vi "dotNET improvments.vi"() -> ()   [LabVIEW 2026]
uses:
  <vilib>/Utility/sysdir.llb/System Directory Type.ctl
  <vilib>/Platform/dotnet.llb/.NET Core Object To Variant.vi
  <vilib>/Platform/dotnet.llb/To .NET Core Object.vi
  C:/Program Files/dotnet/shared/Microsoft.NETCore.App/8.0.24/System.IO.FileSystem.Watcher.dll
  Program Files/dotnet/shared/Microsoft.NETCore.App/8.0.24/System.IO.FileSystem.Watcher.dll
  C:/Program Files/dotnet/shared/Microsoft.NETCore.App/8.0.24/System.Private.CoreLib.dll
  Program Files/dotnet/shared/Microsoft.NETCore.App/8.0.24/System.Private.CoreLib.dll
panel:
  out "element":string
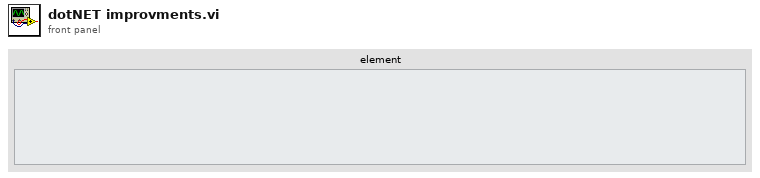
[diagram p1: front panel]
types:
  T1 = typedef "System Directory Type.ctl" = i32
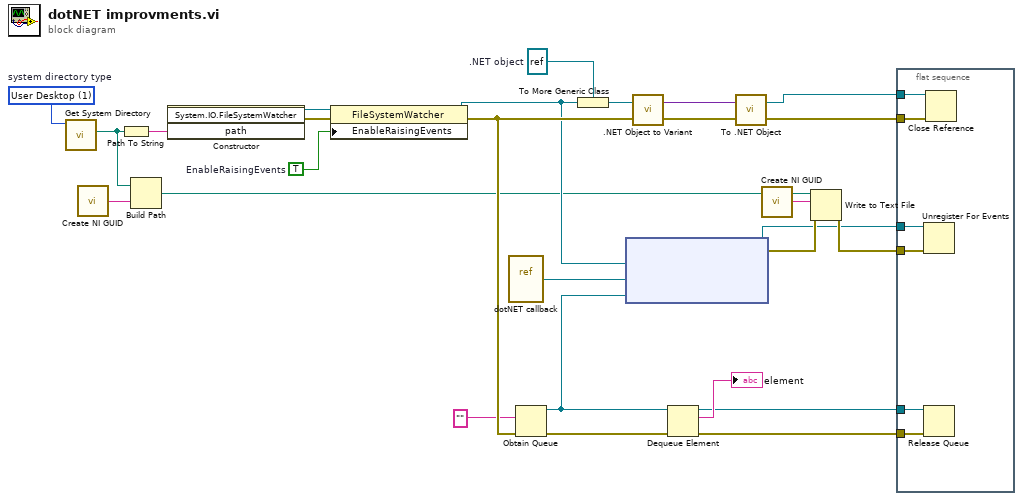
[diagram p0: block diagram]
diagram:
  w12 = refnum<k39> refnum  # .NET object
  w21 = TRUE  # EnableRaisingEvents
  w15 = T1 1 items=["User Home"=0, "User Desktop"=1, "User Documents"=2, "User Application Data"=3, "User Preferences"=4, "User Temporary"=5, "Public Documents"=6, "Public Application Data"=7, "Public Preferences"=8, "Public Cache"=13, "System Core Libraries"=9, "System Installed Libraries"=10, "Application Files"=11, "Boot Volume Root"=12]  # system directory type
  n1 = call <vilib>:"Get System Directory.vi"("system directory type"=w15) -> ("system directory"=w5:path)  [unwired: 10 in]
  n2 = call <vilib>:"Create NI GUID.vi"() -> ("NI GUID"=w6:string)
  n3 = Path To String(path=w5) -> (string=w24:string)
  n4 = Build Path(base path=w5, name or relative path=w6) -> (appended path=w4:path)
  n5 = constructor class="FileSystemWatcher"("path"=w24) -> (reference out=w23:refnum<k39>, error out=w22:errorcluster)  [unwired: 3 in, 2 out]
  n6 = property class="FileSystemWatcher"(reference=w23, error in=w22, "EnableRaisingEvents"=w21) -> (reference out=w13:refnum<k39>, error out=w25:errorcluster)
  n7 = vi-ref "dotNET callback.vi"() -> ("vi reference"=w16:refnum<vi>)
  n8 = Obtain Queue(element data type="", error in (no error)=w25) -> (queue out=w20:refnum<queue>, error out=w18:errorcluster)  [unwired: 3 in, 1 out]
  n9 = To More Generic Class(target class=w12, reference=w13) -> (generic class reference=w11:refnum<k39>)
  n10 = node(w13, w16, w20) -> (w7:refnum<k27>, w26:errorcluster)  [unwired: 2 in]
  n11 = call-poly <vilib>:".NET Object to Variant.vi"("error in (no error)"=w25, ".NET object"=w11) -> ("error out"=w9:errorcluster, "variant"=w14:variant)
  n12 = Dequeue Element(queue=w20, error in (no error)=w18) -> (queue out=w2:refnum<queue>, element=→"element":string, error out=w1:errorcluster)  [unwired: 1 in, 1 out]
  n13 = call-poly <vilib>:"To .NET Object.vi"("error in (no error)"=w9, "anything"=w14) -> ("error out"=w8:errorcluster, ".NET object"=w10:refnum<k39>)
  n14 = call <vilib>:"Create NI GUID.vi"() -> ("NI GUID"=w3:string)
  n15 = Write to Text File(file (use dialog)=w4, text=w3, error in=w26) -> (error out=w27:errorcluster)  [unwired: 1 in, 2 out]
  n16 = flat-sequence {
    tunnel: w27 -> [w31]
    tunnel: w10 -> [w33]
    tunnel: w7 -> [w32]
    tunnel: w8 -> [w30]
    tunnel: w2 -> [w29]
    tunnel: w1 -> [w28]
    frame #0 {
      n17 = Unregister For Events(event registration refnum=w32, error in=w31) -> ()  [unwired: 1 out]
      n18 = Release Queue(queue=w29, error in (no error)=w28) -> ()  [unwired: 1 in, 3 out]
      n19 = Close Reference(reference=w33, error in (no error)=w30) -> ()  [unwired: 1 out]
    }
  }
